vi "Destroy.vi"(0 "reference":refnum<class "AbstractNode.lvclass">, 5 "error in (no error)":errorcluster) -> (14 "reference out":refnum<class "AbstractNode.lvclass">, 19 "error out":errorcluster)   [LabVIEW 2020, in "AbstractNode.lvclass"]
doc: "Destroys an object created with a AbstractNode constructor VI or a subclass of the AbstractNode class. This VI must be reentrant.\n\n[GOOP 2.1]"
uses:
  <resource>/Framework/Providers/Open_GDS/UML/AbstractNode_class/AbstractNode.lvclass
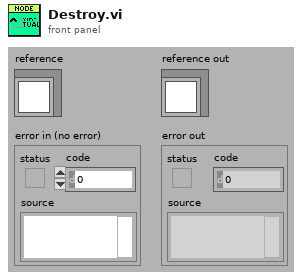
[diagram p1: front panel]
types:
  T1 = typedef "AbstractNode.lvclass/ObjectAttributes.ctl" = cluster{"parent":refnum<class "AbstractNode.lvclass">, "children":refnum<class "AbstractNode.lvclass">[], "Hidden":bool}
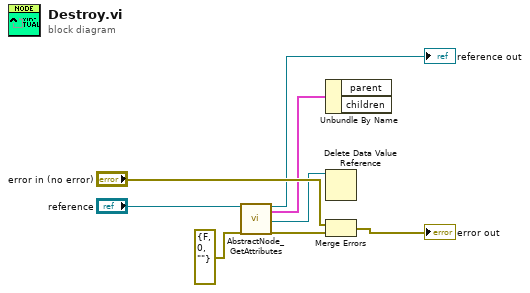
[diagram p0: block diagram]
diagram:
  n1 = call <resource>:"AbstractNode_GetAttributes.vi"("reference in"="reference", "error in (no error)"=errorcluster {"status"=FALSE, "code"=0, "source"=""}) -> ("reference out"=→"reference out":refnum<class "AbstractNode.lvclass">, "Data"=w2:T1, "DataRef"=w1:refnum<data-value>, "error out"=w4:errorcluster)  [unwired: 1 in, 13 out]
  n2 = Unbundle By Name(w2) -> ()  [unwired: 2 out]
  n3 = Delete Data Value Reference(data value reference=w1) -> ()  [unwired: 1 in, 2 out]
  n4 = Merge Errors("error in (no error)", w4) -> (→"error out":errorcluster)
